vi "picoquant_close_device_handle.vi"(8 "error in (no error)":errorcluster, 11 "hydraharp in":refnum<class "hydraharp.lvclass">) -> (0 "error out":errorcluster, 3 "hydraharp out":refnum<class "hydraharp.lvclass">)   [LabVIEW 2015, in "hydraharp.lvclass"]
uses:
  hydraharp.lvclass
  hydraharp.lvclass/hydraharp.ctl
  hhlib.dll
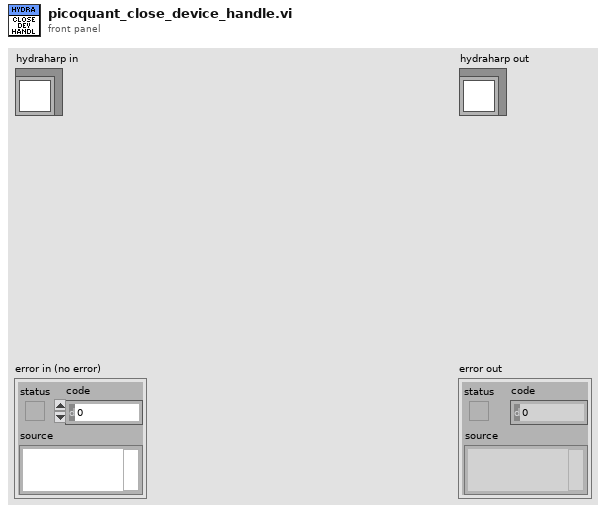
[diagram p1: front panel]
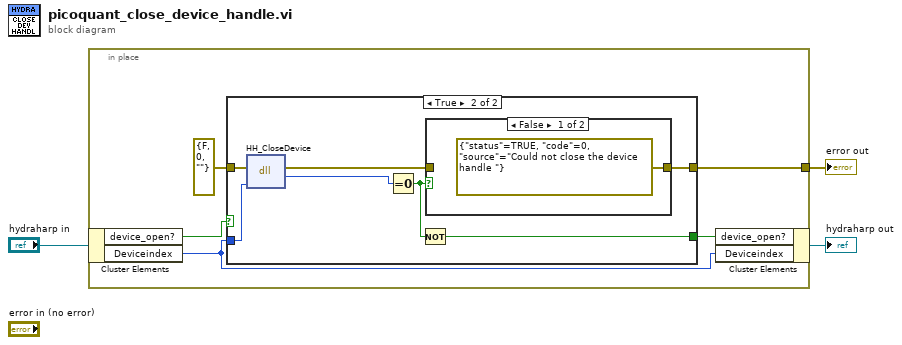
[diagram p0: block diagram]
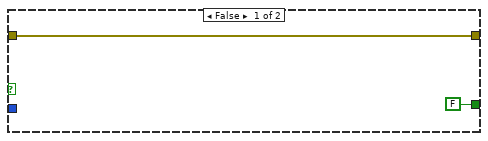
[diagram p2: hidden frame]
diagram:
  n1 = in-place {
    in-place-border: [w6] -> w2
    n2 = in-place-cluster #1("hydraharp in") -> ("device_open?"=w8:bool, "Deviceindex"=w7:i32)
    n3 = case shown="True" w8 {
      tunnel: w7 -> [_ w17]
      tunnel: errorcluster {"status"=FALSE, "code"=0, "source"=""} ("error in (no error)") -> [w10 w16]
      tunnel: [w10 w12] -> w6
      tunnel: [FALSE w15] -> w5
      frame False {
      }
      frame True {
        n4 = dll-call lib="hhlib.dll" fn="HH_CloseDevice"(error in=w16, "devidx"=w17) -> (error out=w13:errorcluster, "return type"=w11:i32)  [unwired: 3 in, 1 out]
        n5 = Equal To 0?(x=w11) -> (x = 0?=w14:bool)
        n6 = Not(x=w14) -> (.not. x?=w15:bool)
        n7 = case shown="False" w14 {
          tunnel: w13 -> [_ w19]
          tunnel: [errorcluster {"status"=TRUE, "code"=0, "source"="Could not close the device handle "} ("error out") w19] -> w12
          frame False {
          }
          frame True {
          }
        }
      }
    }
    n8 = in-place-cluster #1("device_open?"=w5, "Deviceindex"=w7) -> (→"hydraharp out":refnum<class "hydraharp.lvclass">)
  }
  "error out" <- w2
